vi "Set Servo PWM.vi"(8 "error in (no error)":errorcluster, 9 "LEDn (PWM channel)":T1(ring), 10 "Servo Speed (-100 to 100%)":dbl, 11 "LINX-PCA9865 PWM in":refnum<class "LINX-PCA9685 PWM.lvclass">) -> (0 "error out":errorcluster, 3 "LINX-PCA9865 PWM out":refnum<class "LINX-PCA9685 PWM.lvclass">)   [LabVIEW 2020, in "LINX-PCA9685 PWM.lvclass"]
uses:
  LINX-PCA9685 PWM.lvclass
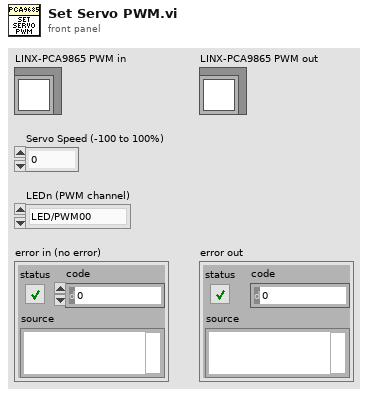
[diagram p1: front panel]
types:
  T1 = enum16{"LED/PWM00", "LED/PWM01", "LED/PWM02", "LED/PWM03", "LED/PWM04", "LED/PWM05", "LED/PWM06", "LED/PWM07", "LED/PWM08", "LED/PWM09", "LED/PWM10", "LED/PWM11", "LED/PWM12", "LED/PWM13", "LED/PWM14", "LED/PWM15"}
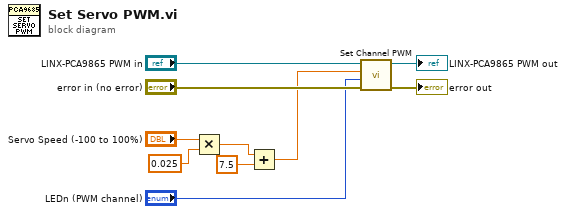
[diagram p0: block diagram]
diagram:
  n1 = Multiply(x="Servo Speed (-100 to 100%)", y=0.025) -> (x*y=w2:dbl)
  n2 = Add(x=w2, y=7.5) -> (x+y=w1:dbl)
  n3 = call-dynamic "Set Channel PWM.vi"("error in (no error)"="error in (no error)", "Channel"="LEDn (PWM channel)", "Duty Cycle 50%)"=w1, "PWM in"="LINX-PCA9865 PWM in") -> ("error out"=→"error out":errorcluster, "PWM out"=→"LINX-PCA9865 PWM out":refnum<class "LINX-PCA9685 PWM.lvclass">)  [unwired: 6 in]
